vi "Create Monitor Log (pcap).vi"(8 "error in":errorcluster, 9 "Timestamp":bool=TRUE, 10 "Name (ARINC664Log.pcap)":string="ARINC664Log.pcap", 11 "Monitor Log Directory and Base FIle (/home/lvuser/)":string="/home/lvuser/afdx_monitor_log") -> (0 "error out":errorcluster, 2 "pcap_dumper_t":u64, 3 "pcap_t out":u64)   [LabVIEW 2020, in "AIM ARINC 664 Engine.lvlib" / "Implementation.lvlib" / "Monitor Execution Unit.lvclass"]
uses:
  Monitor Execution Unit.lvclass
  libpcaplv/libpcaplv.lvlib
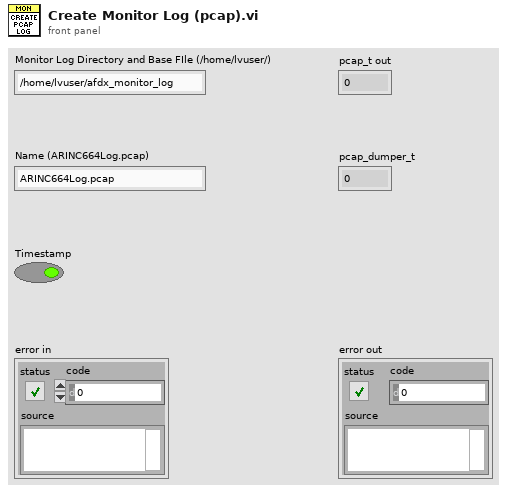
[diagram p1: front panel]
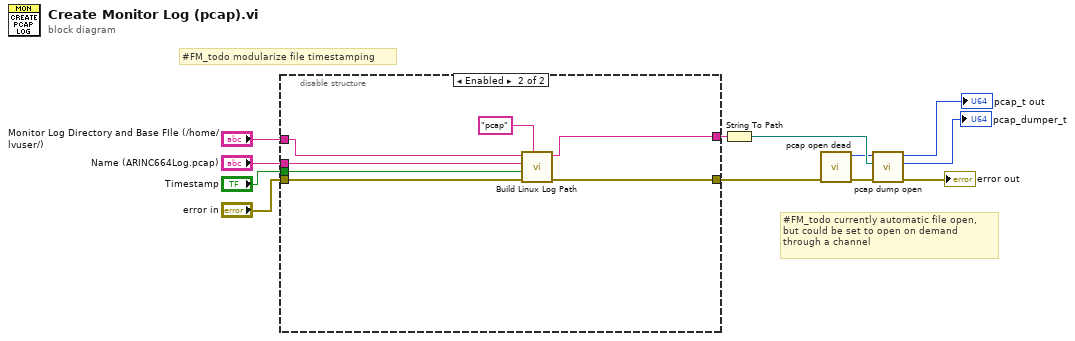
[diagram p0: block diagram]
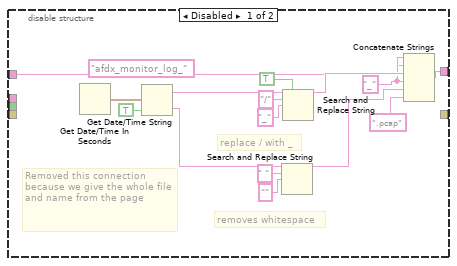
[diagram p2: hidden frame]
diagram:
  # "#FM_todo currently automatic file open,\nbut could be set to open on demand\nthrough a channel"
  # "#FM_todo modularize file timestamping"
  n1 = disable-structure shown="Enabled" {
    disable-tunnel: [w27 w34] -> w12
    disable-tunnel: "Monitor Log Directory and Base FIle (/home/lvuser/)" -> [w14 w33]
    disable-tunnel: "Name (ARINC664Log.pcap)" -> [_ w32]
    disable-tunnel: "error in" -> [_ w31]
    disable-tunnel: [_ w30] -> w2
    disable-tunnel: "Timestamp" -> [_ w29]
    frame Disabled {
      w13 = "_" ("string")
      (unwired) "afdx_monitor_log_" ("string")
      # "Removed this connection because we give the whole file and name from the page"
      # "removes whitespace"
      # "replace / with _"
      n2 = Get Date/Time In Seconds() -> (seconds since 1Jan1904=w26:timestamp)
      n3 = Get Date/Time String(seconds (now)=w26, want seconds? (F)=TRUE) -> (date string=w25:string, time string=w19:string)  [unwired: 1 in]
      n4 = Search and Replace String(input string=w19, search string=" ", replace string="" ("replace string (\"\")")) -> (result string=w18:string)  [unwired: 5 in, 3 out]
      n5 = Search and Replace String(replace all?=TRUE ("replace all? (F)"), input string=w25, search string="/", replace string="_" ("replace string (\"\")")) -> (result string=w24:string)  [unwired: 4 in, 3 out]
      n6 = Concatenate Strings(w14, w13, w24, w13, w18, ".pcap" ("string")) -> (w27:string)
    }
    frame Enabled {
      n7 = call "Build Linux Log Path.vi"("Extension"="pcap", "error in (no error)"=w31, "Timestamp"=w29, "Name"=w32, "Log File Directory"=w33) -> ("error out"=w30:errorcluster, "Log File Path"=w34:string)  [unwired: 5 in]
    }
  }
  n8 = String To Path(string=w12) -> (path=w9:path)
  n9 = call "pcap open dead.vi"("error in"=w2) -> ("error out"=w11:errorcluster, "pcap_t"=w8:u64)  [unwired: 9 in]
  n10 = call "pcap dump open.vi"("error in"=w11, "capture file path"=w9, "pcap_t in"=w8) -> ("error out"=→"error out":errorcluster, "pcap_dumper_t"=→"pcap_dumper_t":u64, "pcap_t out"=→"pcap_t out":u64)  [unwired: 6 in]
